vi "GlobalVariable.vi"() -> ()   [LabVIEW 2019]
panel:
  out "max data":dbl
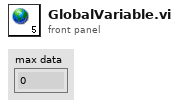
[diagram p1: front panel]
diagram:
